vi "键盘.vi"(1 "关闭":bool, 3 "打开":bool) -> ()   [LabVIEW 2013]
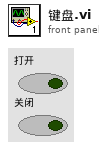
[diagram p1: front panel]
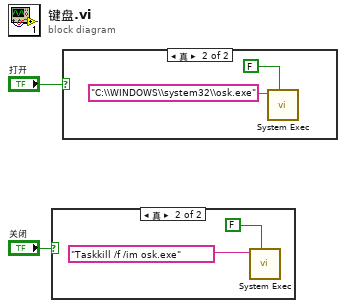
[diagram p0: block diagram]
diagram:
  n1 = case shown="真" "关闭" {
    frame False {
    }
    frame True {
      n2 = call <vilib>:"System Exec.vi"("wait until completion? (T)"=FALSE, "command line"="Taskkill /f /im osk.exe") -> ()  [unwired: 6 in, 4 out]
    }
  }
  n3 = case shown="真" "打开" {
    frame False {
    }
    frame True {
      n4 = call <vilib>:"System Exec.vi"("wait until completion? (T)"=FALSE, "command line"="C:\\WINDOWS\\system32\\osk.exe") -> ()  [unwired: 6 in, 4 out]
    }
  }
